vi "Dashboard Main.vi"() -> ()   [LabVIEW 2013]
uses:
  TargetType.ctl
  <vilib>/event_ctls.llb/eventvkey.ctl
  <vilib>/Rock Robotics/WPI/Dashboard/WPI_DashboardLogging Global.vi
  <vilib>/Utility/config.llb/Write Key (String).vi
  <vilib>/Utility/config.llb/Write Key (I32).vi
  <vilib>/Utility/config.llb/NI_LVConfig.lvlib
panel:
  in  "Camera Settings":T1={"Frame Rate"=30, "Compression"=30, "Size"=1} {"Frame Rate" scale=1.0..30.0; "Size" items=["640x480", "320x240", "160x120"]}
  out "Image 3":T2(plugin-control)
  out "Target Info 2":T4(array[cluster])
  in  "Instructions: 3":string="Images:\nUse the tab immediately below to choose the image source. Update the camera settings or the image directory so that you have images or video to test with.\n\nCalibration:\nYou can update Color Component ranges directly, or by clicking and drawing a line on the colored strip in the Image control. The Std Dev multipliers and where the strip is drawn determine the calibration values.\n\nUse Debugging tab to view the result of the color range threshold .\n\nArea Size LImit is used to ignore objects too small or far away to care about.\n\nThe Details tab contains score details for each target and subObject.\n\nCamera Type is used to select lens angles for distance calculation.\n\nVertical strips with no adjacent horizontal strip are identified as \"not hot\" and marked in blue.\nThe numeric scores indicate represent aspect ratio and rectangularity.\n\nWhen both strips are near enough, the pair is identified as \"hot\" and marked in green. Scores\nindicate the left, right, ratio of widths, and vertical positioning.\n\nAny score that falls below cutoff is drawn in red and bounding box is drawn in red."
  in  "Instructions:":string="Images:\nUse the tab immediately below to choose the image source. Update the camera settings or the image directory so that you have images or video to test with.\n\nCalibration:\nYou can update Color Component ranges directly, or by clicking and drawing a line on the colored strip in the Image control. The Std Dev multipliers and where the strip is drawn determine the calibration values.\n\nUse Debugging tab to view the result of the color range threshold .\n\nArea Size LImit is used to ignore objects too small or far away to care about.\n\nThe Details tab contains score details for each target and subObject.\n\nCamera Type is used to select lens angles for distance calculation.\n\nVertical strips with no adjacent horizontal strip are identified as \"not hot\" and marked in blue.\nThe numeric scores indicate represent aspect ratio and rectangularity.\n\nWhen both strips are near enough, the pair is identified as \"hot\" and marked in green. Scores\nindicate the left, right, ratio of widths, and vertical positioning.\n\nAny score that falls below cutoff is drawn in red and bounding box is drawn in red."
  out "Image 2":T2(plugin-control)
  out "Image Message":string="Timeout in Camera Communications"
  in  "Rec Mode":enum32{"Stop", "Record", "Playback"}(radio)
  in  "Dashboard Tab":T5(tab)
  out "MotorSliders R":cluster{"MotorSlide1":dbl, "MotorSlide2":dbl} {"MotorSlide2" scale=-1.0..1.0 scale format="%#_2e"; "MotorSlide1" scale=-1.0..1.0 scale format="%#_2e"}
  out "MotorChart R":cluster{"Numeric":dbl, "Numeric":dbl}(graph)
  out "MotorSliders L":T6 {"MotorSlide4 2" scale=0.0..14.0 scale format="%#_2e"; "MotorSlide2" scale=-1.0..1.0 scale format="%#_2e"; "MotorSlide1" scale=-1.0..1.0 scale format="%#_2e"}
  out "MotorChart L":T7(graph)
  out "JS1 Z":dbl(slide) scale=-1.0..1.0 scale format="%#_2e"
  out "Joystick 1":cluster{"X":dbl, "Y":dbl}[](graph)
  out "JS Buttons 1":T8
  out "JS2 Z":dbl(slide) scale=-1.0..1.0 scale format="%#_2e"
  out "Joystick 2":cluster{"X":dbl, "Y":dbl}[](graph)
  out "JS Buttons 2":T8
  out "Mode":T9(ring)=enum."Auto Disabled"
  out "Camera IP":string
  in  "DB Camera Config":bool
  out "fps":dbl format="%#.1g"
  out "Mbps":dbl format="%#.1g"
  out "Mbps 2":bool
  out "Mask 4":T2(plugin-control)
  out "Goal Hot Or Not?":bool
  in  "Enable":bool
  in  "Color Components":T10={"Hue"={61.0, 119.0}, "Sat"={55.0, 255.0}, "Val"={64.0, 243.0}} {"Val" scale=0.0..255.0; "Sat" scale=0.0..255.0; "Hue" scale=0.0..255.0 scale format="%#_3g"}
  in  "Score Cutoff":dbl(slide)=38.3177570093458 scale=0.0..100.0
  in  "Camera Type":enum16{"206", "1011", "1013"}(ring)=enum."1013"
  in  "Area Size Limit %":dbl=0.06 format="%#_13g"
  in  "Std Devs":cluster{"Hue":dbl, "Sat":dbl, "Val":dbl}={"Hue"=4.0, "Sat"=6.0, "Val"=4.0}
  in  "milliseconds to wait":u32=400
  in  "Auton Routine Names":string[](array[string])
  in  "Routine selected":u16(ring)
  in  "Test Slider":dbl(slide) scale=0.0..100.0 scale format="%#_3g"
  in  "On/Off":bool caption="Solenoid"
  in  "Test Name":u16(ring) items=["Select the test to run...", "Example Test", "-------------------------------", "List of tests is built in robot code.", "Replace with your own automated tests."]
  in  "Test Tree":string(tree)
  in  "Motor":cluster{"Value":dbl, "Enable":bool} {"Value" scale=-1.0..1.0 scale format="%#_3g"}
  out "Progress":T11 {"Test Progress" scale=0.0..100.0}
  in  "Rev/Fwd":cluster{"Forward":bool, "Reverse":bool}
  in  "Test Ring":u16(ring) items=["Auto", "Fixed indoor", "Fixed outdoor 1", "Fixed outdoor 2", "Fixed fluorescent 1", "Fixed fluorescent 2", "Hold current"]
  in  "Listbox":i32(listbox)
  out "Tree":string(tree)
  # "Left"
  # "Front"
  # "Right"
  # "Battery"
  # "Customize by placing controls and indicators here and name to\nmatch Dashboard Variables on robot."
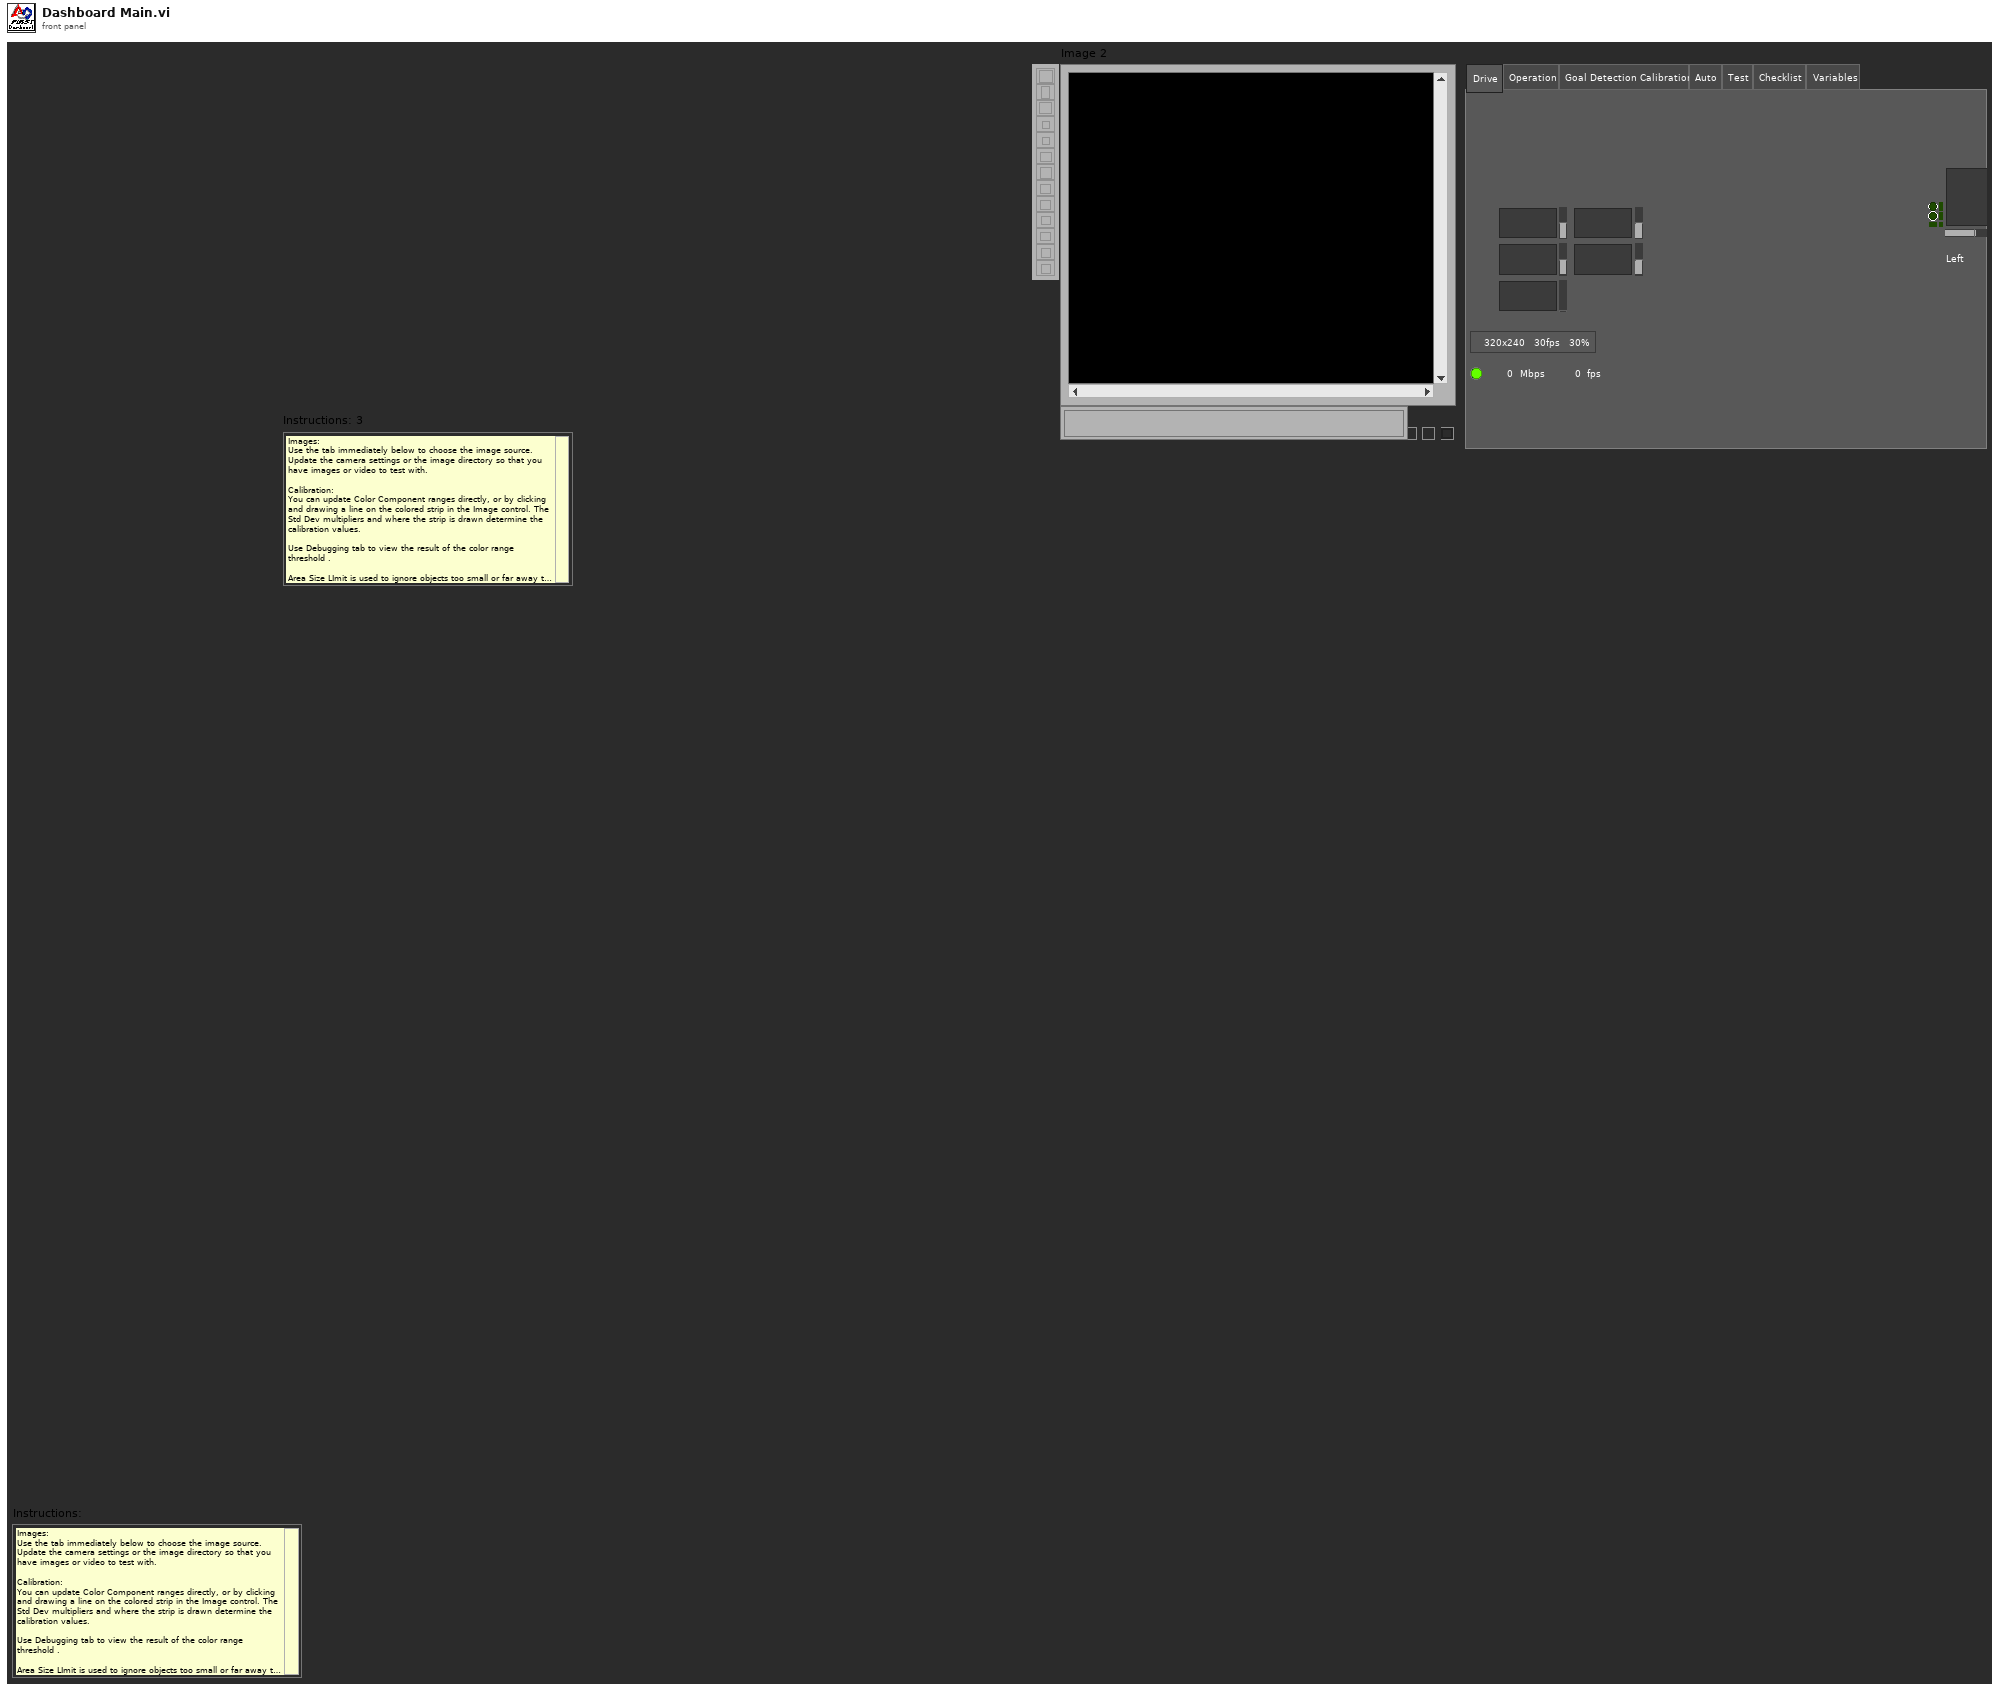
[diagram p1: front panel]
types:
  T1 = cluster{"Frame Rate":i32, "Compression":i32, "Size":u16}
  T2 = typedef "IMAQ Image.ctl" = refnum<image>
  T3 = typedef "TargetType.ctl" = enum16{"Not Hot", "Hot"}
  T4 = cluster{"Scores":cluster{"Total":dbl, "Left":dbl, "Right":dbl, "Ratio":dbl, "Vertical":dbl, "index":i32, "State":T3}, "Verticals":cluster{"Horizontal?":bool, "Aspect Score":dbl, "Rect Score":dbl, cluster{"Left":dbl, "Top":dbl, "Right":dbl, "Bottom":dbl}, "Equiv H":dbl, "Equiv V":dbl}, "Horizontals":cluster{"Horizontal?":bool, "Aspect Score":dbl, "Rect Score":dbl, cluster{"Left":dbl, "Top":dbl, "Right":dbl, "Bottom":dbl}, "Equiv H":dbl, "Equiv V":dbl}, "Distance ft":dbl, "Center":cluster{"X":dbl, "Y":dbl}}[]
  T5 = enum32{"Drive", "Operation", "Goal Detection Calibration", "Auto", "Test", "Checklist", "Variables"}
  T6 = cluster{"MotorSlide1":dbl, "MotorSlide2":dbl, "MotorSlide4 2":dbl}
  T7 = cluster{"Numeric":dbl, "Numeric":dbl, "Battery":sgl}
  T8 = cluster{bool, bool, bool, bool, bool, bool, bool, bool, bool, bool, bool, bool}
  T9 = enum8{"Tele-Op Disabled", "Tele-Op Enabled", "Auto Disabled", "Auto Enabled", "Test Disabled", "Test Enabled", ""}
  T10 = cluster{"Hue":cluster{dbl, dbl}, "Sat":cluster{dbl, dbl}, "Val":cluster{dbl, dbl}}
  T11 = cluster{"Test Progress":u8, "Test Progress Text":string}
  T12 = enum32{"Drive", "Operation", "Vision", "Auto", "Test", "Checklist", "Variables"}
  T13 = typedef "Image Type" = u32
  T14 = cluster{"Horizontal":bool, "Aspect Score":dbl, "Rect Score":dbl, cluster{"Left":dbl, "Top":dbl, "Right":dbl, "Bottom":dbl}, "Equiv H":dbl, "Equiv V":dbl}[]
  T15 = cluster{cluster{dbl, dbl}, cluster{dbl, dbl}, cluster{dbl, dbl}}
  T16 = cluster{"Scores":cluster{"Total":dbl, "Left":dbl, "Right":dbl, "Ratio":dbl, "Vertical":dbl, "index":i32, "State":T3}, "Verticals":cluster{"Horizontal?":bool, "Aspect Score":dbl, "Rect Score":dbl, cluster{"Left":dbl, "Top":dbl, "Right":dbl, "Bottom":dbl}, "Equiv H":dbl, "Equiv V":dbl}, "Horizontals":cluster{"Horizontal?":bool, "Aspect Score":dbl, "Rect Score":dbl, cluster{"Left":dbl, "Top":dbl, "Right":dbl, "Bottom":dbl}, "Equiv H":dbl, "Equiv V":dbl}, "Validated":bool}[]
  T17 = cluster{"Scores":cluster{"Total":dbl, "Left":dbl, "Right":dbl, "Ratio":dbl, "Vertical":dbl, "index":i32, "State":T3}, "Verticals":cluster{"Horizontal?":bool, "Aspect Score":dbl, "Rect Score":dbl, cluster{"Left":dbl, "Top":dbl, "Right":dbl, "Bottom":dbl}, "Equiv H":dbl, "Equiv V":dbl}, "Horizontals":cluster{"Horizontal?":bool, "Aspect Score":dbl, "Rect Score":dbl, cluster{"Left":dbl, "Top":dbl, "Right":dbl, "Bottom":dbl}, "Equiv H":dbl, "Equiv V":dbl}, "Distance (ft)":dbl, "Target Center (-1 to 1)":cluster{"X":dbl, "Y":dbl}}[]
  T18 = cluster{"Scores":cluster{"Total":dbl, "Left":dbl, "Right":dbl, "Ratio":dbl, "Vertical":dbl, "index":i32, "State":T3}, "Verticals":cluster{"Horizontal?":bool, "Aspect Score":dbl, "Rect Score":dbl, cluster{"Left":dbl, "Top":dbl, "Right":dbl, "Bottom":dbl}, "Equiv H":dbl, "Equiv V":dbl}, "Horizontals":cluster{"Horizontal?":bool, "Aspect Score":dbl, "Rect Score":dbl, cluster{"Left":dbl, "Top":dbl, "Right":dbl, "Bottom":dbl}, "Equiv H":dbl, "Equiv V":dbl}, "Distance (ft)":dbl, "Target Center (-1 to 1)":cluster{"X":dbl, "Y":dbl}}
  T19 = typedef "NI_LVConfig.lvlib/Config Data RefNum.ctl" = refnum<k1>
  T20 = cluster{"Digital Inputs":bool[], "Digital Outputs":bool[]}
  T21 = cluster{"Competition mode":bool, "Robot Link":bool, "Autonomous":bool, "Enabled":bool, "E-Stop":bool, "Simulated":bool, "TestMode":bool, "Docked Window":bool}
  T22 = cluster{"Boolean Array[0]":bool, "Boolean Array[1]":bool, "Boolean Array[2]":bool, "Boolean Array[3]":bool, "Boolean Array[4]":bool, "Boolean Array[5]":bool, "Boolean Array[6]":bool, "Boolean Array[7]":bool, "Boolean Array[8]":bool, "Boolean Array[9]":bool, "Boolean Array[10]":bool, "Boolean Array[11]":bool}
  T23 = typedef "eventvkey.ctl" = enum16{"ASCII", "Enter", "Return", "Shift", "Ctrl", "Alt", "Cmd", "Opt", "Caps", "NumLock", "Clear", "Break", "Up", "Down", "Left", "Right", "Insert", "Delete", "Home", "End", "PageUp", "PageDown", "Escape", "Help", "Pause", "ScrollLock", "F1", "F2", "F3", "F4", "F5", "F6", "F7", "F8", "F9", "F10", "F11", "F12", "F13", "F14", "F15", "F16", "F17", "F18", "F19", "F20", "F21", "F22", "F23", "F24", "Play", "VolumeUp", "VolumeDown", "Mute", "Two Byte Char"}
  T24 = cluster{"Image Size":bool, "Image Type":bool, "Pixel Value":bool, "ROI Information":bool, "Zoom Factor":bool}
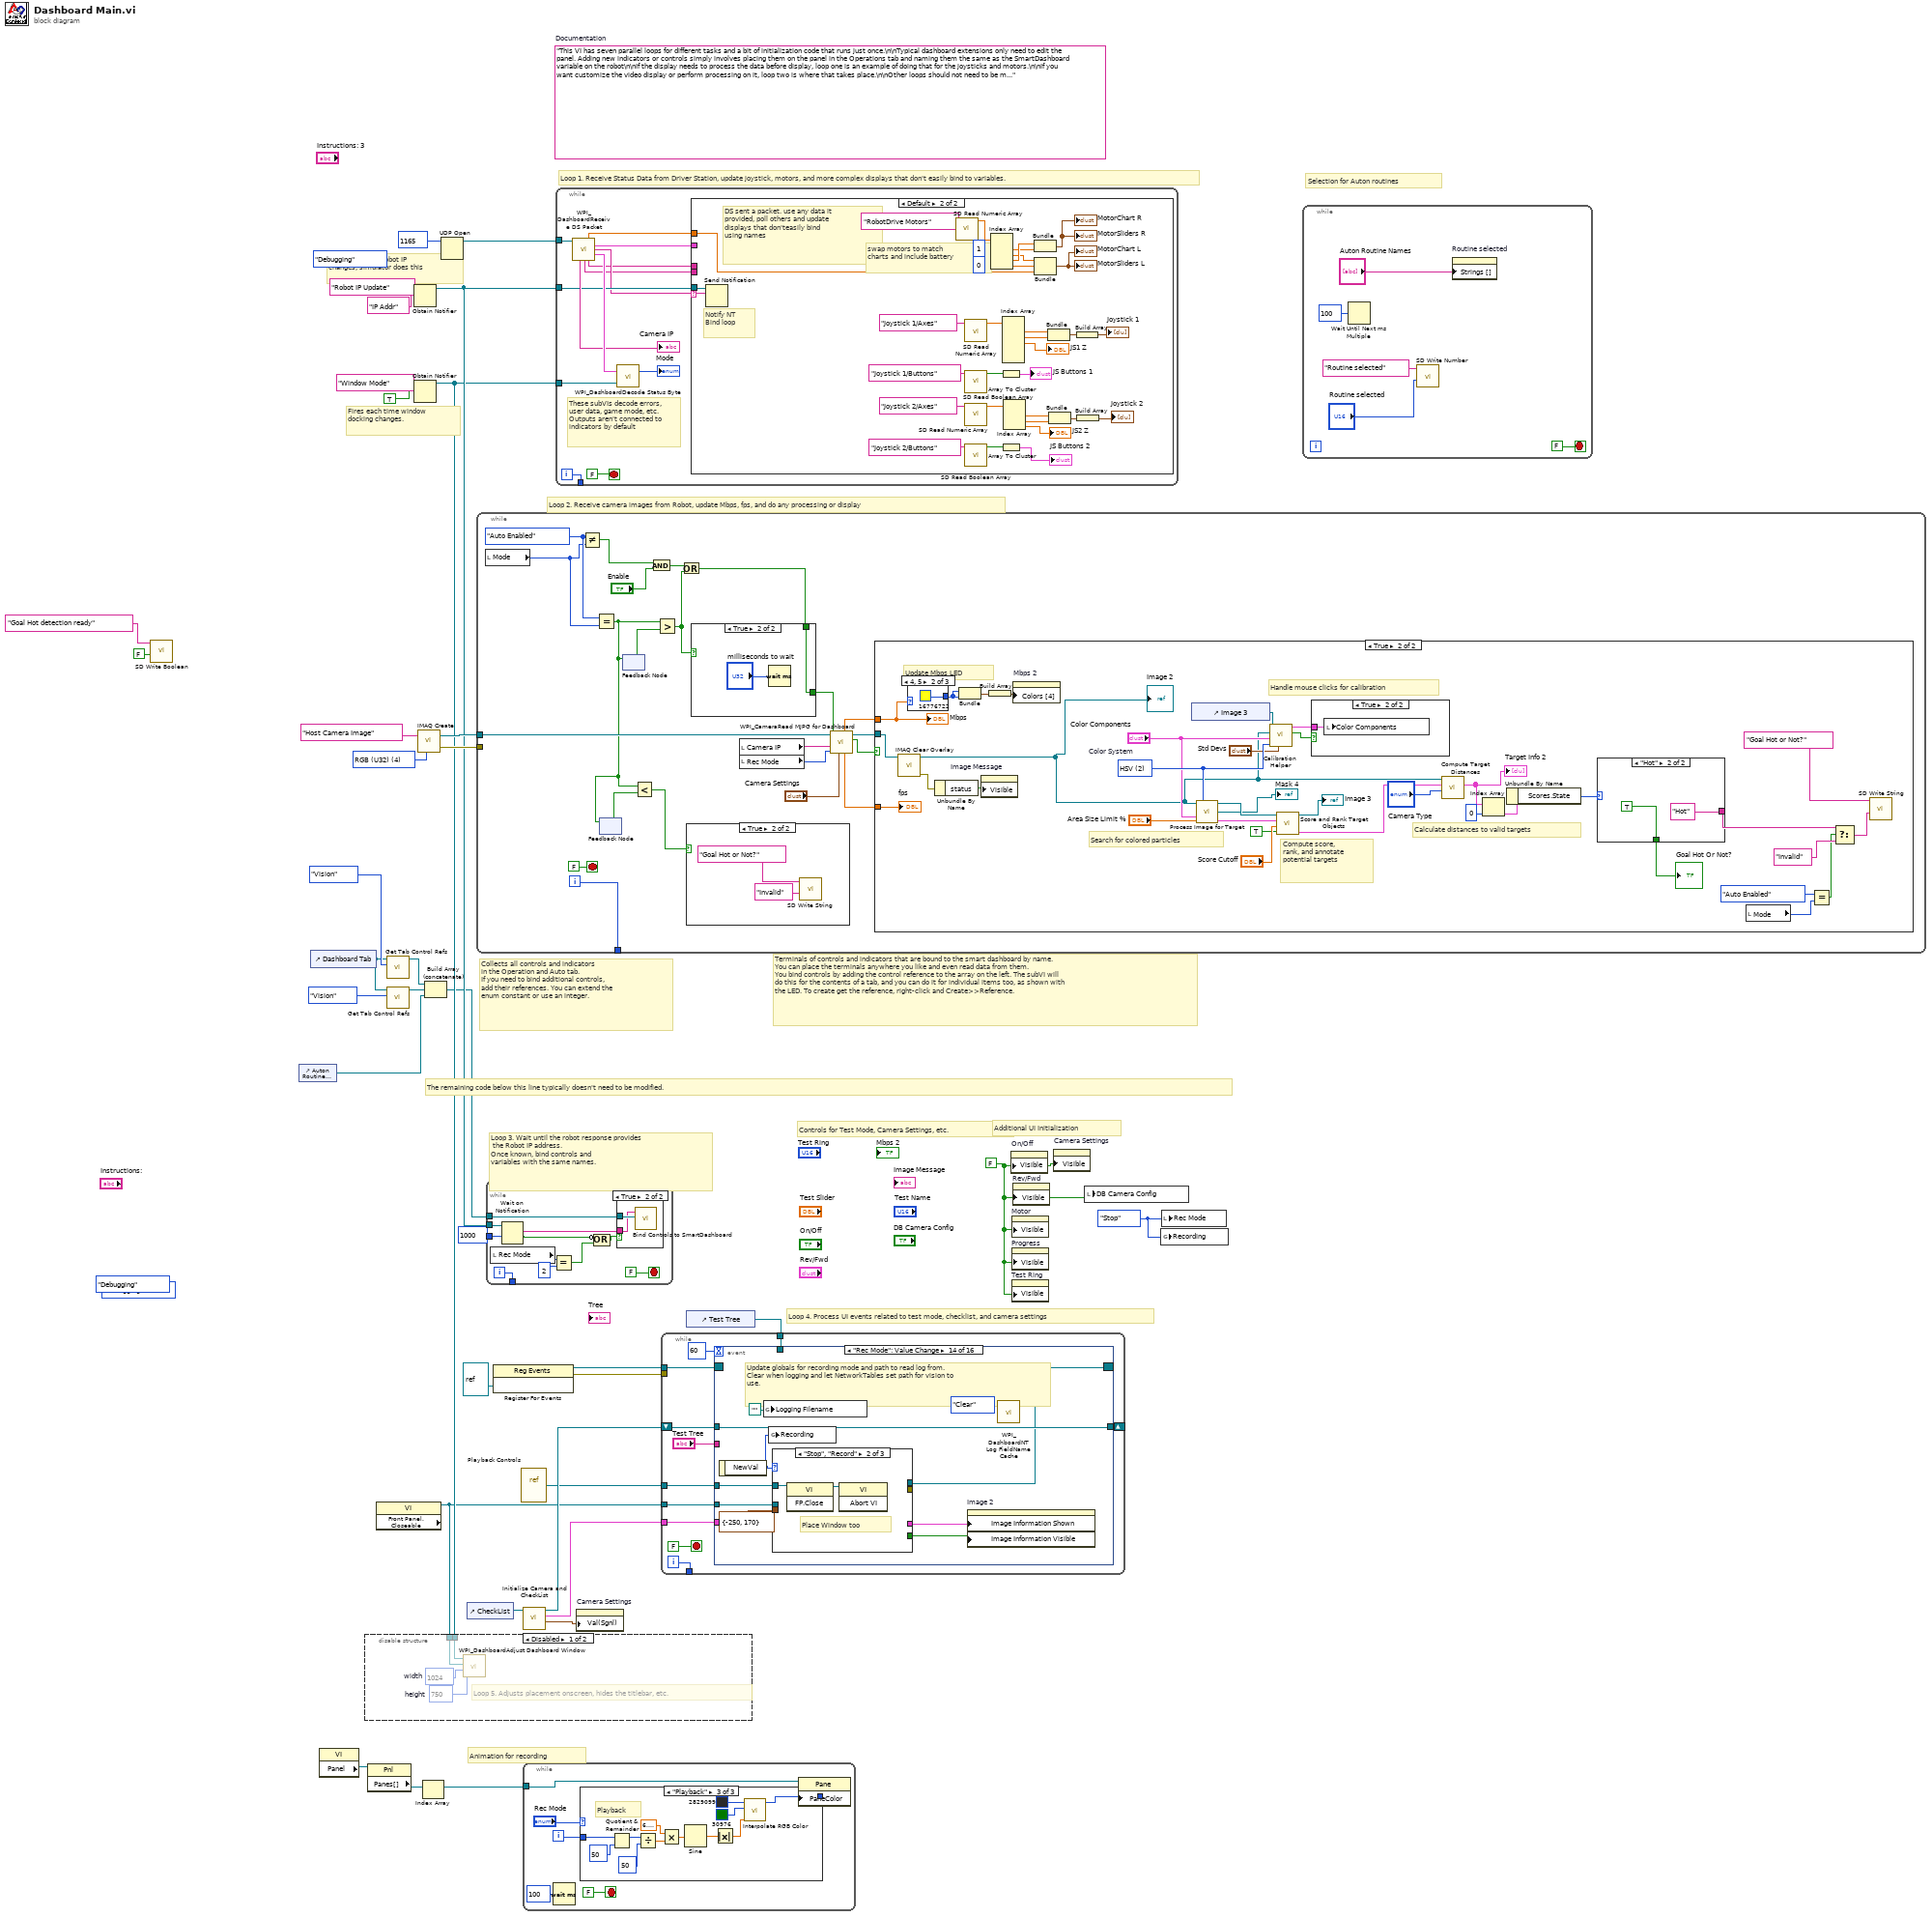
[diagram p0: block diagram]
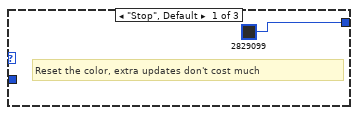
[diagram p3: hidden frame]
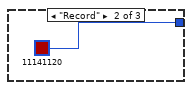
[diagram p4: hidden frame]
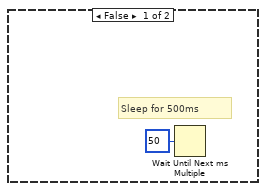
[diagram p8: hidden frame]
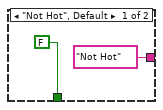
[diagram p9: hidden frame]
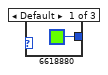
[diagram p11: hidden frame]
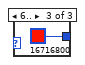
[diagram p12: hidden frame]
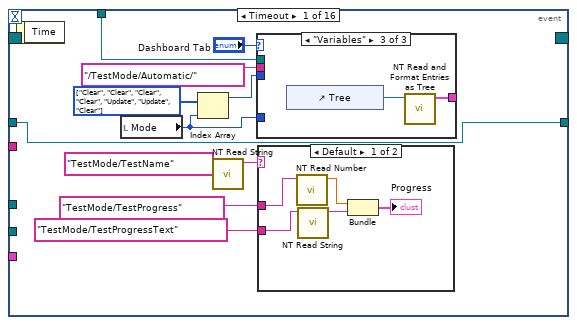
[diagram p13: hidden frame]
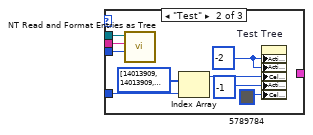
[diagram p15: hidden frame]
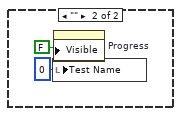
[diagram p16: hidden frame]
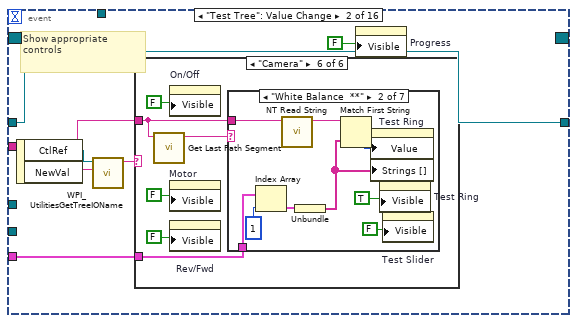
[diagram p17: hidden frame]
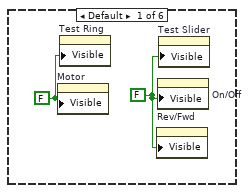
[diagram p18: hidden frame]
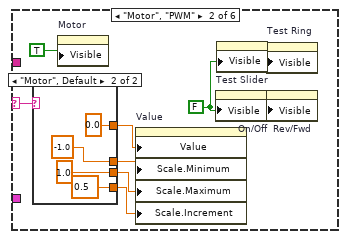
[diagram p19: hidden frame]
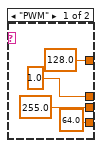
[diagram p20: hidden frame]
diagram:
  (unwired) enum32{"Debugging", "Details"}."Debugging" ("Tabbed Info")
  (unwired) enum32{"Debugging", "Details"}."Debugging" ("Tabbed Info")
  (unwired) enum32{"Debugging", "Details"}."Debugging" ("Tabbed Info")
  w10 = enum32{"Stop", "Record", "Playback"}."Stop" ("Rec Mode")
  w25 = FALSE ("Visible")
  (unwired) "This VI has seven parallel loops for different tasks and a bit of initialization code that runs just once.\n\nTypical dashboard extensions only need to edit the panel. Adding new indicators or controls simply involves placing them on the panel in the Operations tab and naming them the same as the SmartDashboard variable on the robot\n\nIf the display needs to process the data before display, loop one is an example of doing that for the joysticks and motors.\n\nIf you want customize the video display or perform processing on it, loop two is where that takes place.\n\nOther loops should not need to be modified. They are pretty standard, and document the task they perform."  # Documentation
  w35 = T13 4 items=["Grayscale (U8)", "Grayscale (I16)", "Grayscale (SGL)", "Complex (CSG)", "RGB (U32)", "HSL (U32)", "RGB (U64)"] ("Image Type")
  # "Selection for Auton routines"
  # "Controls for Test Mode, Camera Settings, etc."
  # "Additional UI Initialization"
  # "Animation for recording"
  # "Fires each time robot IP\nchanges, simulator does this"
  # "Fires each time window\ndocking changes."
  # "Collects all controls and indicators\nin the Operation and Auto tab.\nIf you need to bind additional controls,\nadd their references. You can extend the\nenum constant or use an integer."
  # "The remaining code below this line typically doesn't need to be modified."
  # "Loop 4. Process UI events related to test mode, checklist, and camera settings"
  # "Terminals of controls and indicators that are bound to the smart dashboard by name.\nYou can place the terminals anywhere you like and even read data from them.\nYou bind controls by adding the control reference to the array on the left. The subVI will\ndo this for the contents of a tab, and you can do it for individual items too, as shown with\nthe LED. To create get the reference, right-click and Create>>Reference."
  # "Loop 3. Wait until the robot response provides\n the Robot IP address.\nOnce known, bind controls and\nvariables with the same names."
  # "Loop 1. Receive Status Data from Driver Station, update joystick, motors, and more complex displays that don't easily bind to variables."
  # "Loop 2. Receive camera images from Robot, update Mbps, fps, and do any processing or display"
  n1 = call <vilib>:"SD Write Boolean.vi"("Boolean"=FALSE, "Name"="Goal Hot detection ready") -> ()  [unwired: 8 in, 2 out]
  n2 = control-ref of="Auton Routine Names"() -> (w3:refnum<vi>)
  n3 = control-ref of="Dashboard Tab"() -> (w8:refnum<vi>)
  n4 = property class="VI"() -> ("Panel"=w19:refnum<vi>)  [unwired: 2 in, 2 out]
  n5 = property class="Pnl"(reference=w19) -> ("Panes[]"=w20:refnum<vi>[])  [unwired: 1 in, 2 out]
  n6 = property class="VI" props=["Front Panel.Closeable"]() -> (reference out=w9:refnum<vi>)  [unwired: 2 in, 2 out]
  n7 = call <vilib>:"Get Tab Control Refs.vi"("Page Index"=T12."Vision" ("Dashboard Tab"), "TabControl in"=w8) -> ("ControlsOnPage"=w6:refnum<vi>[])  [unwired: 9 in]
  n8 = call <vilib>:"Get Tab Control Refs.vi"("Page Index"=T12."Vision" ("Dashboard Tab"), "TabControl in"=w8) -> ("ControlsOnPage"=w7:refnum<vi>[])  [unwired: 9 in]
  n9 = Obtain Notifier(name (unnamed)="Robot IP Update", notification data type="IP Addr" ("name (unnamed)")) -> (notifier out=w29:refnum<notifier>)  [unwired: 2 in, 2 out]
  n10 = Obtain Notifier(name (unnamed)="Window Mode", notification data type=TRUE) -> (notifier out=w12:refnum<notifier>)  [unwired: 2 in, 2 out]
  n11 = disable-structure shown="Disabled" {
    disable-tunnel: w12 -> [w39 _]
    disable-tunnel: w9 -> [w38 _]
    frame Disabled {
      w40 = 750  # height
      w41 = 1024  # width
      # "Loop 5. Adjusts placement onscreen, hides the titlebar, etc."
      n12 = call <vilib>:"WPI_DashboardAdjust Dashboard Window.vi"("height"=w40, "width"=w41, "reference in"=w38, "Notifier in"=w39) -> ()  [unwired: 8 in]
    }
    frame Enabled {
    }
  }
  n13 = call "IMAQ Create"("Image Name"="Host Camera Image", "Image Type"=w35) -> ("New Image"=w33:T2, "error out"=w32:errorcluster)  [unwired: 2 in, 1 out]
  n14 = Index Array(array=w20) -> (element=w18:refnum<vi>)  [unwired: 1 in]
  n15 = Build Array (concatenate)(w6, w7, w3) -> (w5:refnum<vi>[])
  n16 = UDP Open(11:u16 1165 ("port")) -> (port=w36:refnum<k16>)  [unwired: 2 in, 4 out]
  n17 = control-ref of="CheckList"() -> (w11:refnum<vi>)
  n18 = while {
    tunnel: w33 -> [w51]
    tunnel: w32 -> [_]
    tunnel: [w62] -> _
    i -> [w62]
    stop <- FALSE stop-if-true
    w50 = T9."Auto Enabled" ("x")
    n19 = local read "Mode"() -> (w49:T9)
    n20 = Not Equal?(x=w50, y=w49) -> (x != y?=w53:bool)
    n21 = Equal?(x=w50, y=w49) -> (x = y?=w43:bool)
    n22 = feedback #1() -> (w44:bool)  [unwired: 1 in]
    n23 = feedback-in #1(w43) -> ()
    n24 = feedback-in #2(w43) -> ()
    n25 = feedback #2() -> (w48:bool)  [unwired: 1 in]
    n26 = Less?(x=w43, y=w44) -> (x < y?=w42:bool)
    n27 = And(x=w53, y="Enable") -> (x .and. y?=w52:bool)
    n28 = Greater?(x=w43, y=w48) -> (0:w47:bool)
    n29 = Or(x=w52, y=w47) -> (x .or. y?=w45:bool)
    n30 = case shown="True" w42 {
      frame False {
      }
      frame True {
        n31 = call <vilib>:"SD Write String.vi"("String"="Invalid", "Name"="Goal Hot or Not?") -> ()  [unwired: 8 in, 2 out]
      }
    }
    n32 = case shown="True" w47 {
      tunnel: [w66 w67] -> w46
      tunnel: w45 -> [w66 w67]
      frame False {
      }
      frame True {
        n33 = Wait (ms)(milliseconds to wait="milliseconds to wait") -> ()  [unwired: 1 out]
      }
    }
    n34 = local read "Camera IP"() -> (w55:string)
    n35 = local read "Rec Mode"() -> (w56:enum32{"Stop", "Record", "Playback"})
    n36 = call <vilib>:"WPI_CameraRead MJPG for Dashboard.vi"("Camera Settings"="Camera Settings", "Rec Mode"=w56, "Camera IP"=w55, "Enable"=w46, "Refnum in"=w51) -> ("Active"=w60:bool, "Refnum out"=w61:T2, "FPS"=w59:dbl, "Bandwidth (Mbps)"=w58:dbl)  [unwired: 3 in]
    n37 = case shown="True" w60 {
      tunnel: w61 -> [_ w100]
      tunnel: w58 -> [_ w99]
      tunnel: w59 -> [_ w98]
      frame False {
        # "Sleep for 500ms"
        n38 = Wait Until Next ms Multiple(millisecond multiple=u32 50) -> ()  [unwired: 1 out]
      }
      frame True {
        w91 = u16 2 items=["RGB", "HSL", "HSV", "HSI"]  # Color System
        # "Calculate distances to valid targets"
        # "Search for colored particles"
        # "Handle mouse clicks for calibration"
        # "Compute score,\nrank, and annotate\npotential targets"
        # "Update Mbps LED"
        n39 = call "IMAQ Clear Overlay"("Image"=w100) -> ("error out"=w104:errorcluster, "Image Out"=w82:T2)  [unwired: 2 in, 7 out]
        "Image 2" <- w82
        n40 = case shown="4, 5" w99 {
          tunnel: [u32 6618880 ("Color Box") u32 16776722 ("Color Box") u32 16716800 ("Color Box")] -> w101
          frame Default {
          }
          frame 4, 5 {
          }
          frame 6.. {
          }
        }
        n41 = Unbundle By Name(w104) -> ("status"=w105:bool)
        n42 = Bundle("Color Box"=w101, "Color Box"=w101) -> (w103:cluster{"Color Box":u32, "Color Box":u32})  [unwired: 1 out]
        n43 = property on="Image Message" class="Str"("Visible"=w105) -> ()  [unwired: 2 in, 2 out]
        n44 = Build Array(w103) -> (w102:cluster{"Color Box":u32, "Color Box":u32}[])
        n45 = property on="Mbps 2" class="Bool (strict)"("Colors [4]"=w102) -> ()  [unwired: 2 in, 2 out]
        n46 = control-ref of="Image 3"() -> (w79:refnum<vi>)
        n47 = call "Process Image for Target.vi"("Src Image"=w82, "Color Mode"=w91, "Color Components"="Color Components", "Area Cutoff %"="Area Size Limit %") -> ("Src Image Out"=w96:T2, "Threshold"=→"Mask 4":T2, "Particles"=w94:T14)  [unwired: 9 in]
        n48 = call "Calibration Helper.vi"("Std Devs"="Std Devs", "Color Mode"=w91, "Color Components"="Color Components", "Image"=w82, "Image Ctl Refnum"=w79) -> ("Changed"=w87:bool, "output color"=w89:T15)  [unwired: 5 in]
        n49 = call "Score and Rank Target Objects.vi"("Annotate"=TRUE, "Score Limit"="Score Cutoff", "Particles"=w94, "Image in"=w96) -> ("Target Info"=w93:T16, "Annotated Image"=→"Image 3":T2)  [unwired: 6 in]
        n50 = case shown="True" w87 {
          tunnel: w89 -> [_ w110]
          frame False {
          }
          frame True {
            n51 = local write "Color Components"(w110) -> ()
          }
        }
        n52 = call "Compute Target Distances.vi"("Camera Type"="Camera Type", "Target Info"=w93, "Image in"=w82) -> ("Target Info"=w80:T17)  [unwired: 6 in, 2 out]
        "Target Info 2" <- w80
        n53 = Index Array(array=w80, index=0) -> (element=w84:T18)
        n54 = Unbundle By Name(w84) -> ("Scores.State"=w83:T3)
        n55 = case shown="\"Hot\"" w83 {
          tunnel: [FALSE TRUE] -> w76
          tunnel: ["Not Hot" "Hot"] -> w75
          frame "Not Hot", Default {
          }
          frame "Hot" {
          }
        }
        "Goal Hot Or Not?" <- w76
        n56 = local read "Mode"() -> (w72:T9)
        n57 = Equal?(x=T9."Auto Enabled", y=w72) -> (x = y?=w70:bool)
        n58 = Select(t=w75, s=w70, f="Invalid") -> (s? t:f=w74:string)
        n59 = call <vilib>:"SD Write String.vi"("String"=w74, "Name"="Goal Hot or Not?") -> ()  [unwired: 8 in, 2 out]
        "Mbps" <- w99
        "fps" <- w98
      }
    }
  }
  n60 = while {
    tunnel: w5 -> [w124]
    tunnel: w29 -> [w122]
    tunnel: [w120] -> _
    tunnel: u32 1000 ("milliseconds to wait") -> [w119]
    i -> [w120]
    stop <- FALSE stop-if-true
    n61 = local read "Rec Mode"() -> (w115:enum32{"Stop", "Record", "Playback"})
    n62 = Wait on Notification(notifier=w122, timeout in ms (-1)=w119) -> (notification=w121:string, timed out?=w117:bool)  [unwired: 2 in, 2 out]
    n63 = Equal?(x=w115, y=u16 2 ("Rec Mode")) -> (x = y?=w116:bool)
    n64 = Compound Arithmetic op=OR(invert w117, w116) -> (w118:bool)
    n65 = case shown="True" w118 {
      tunnel: w124 -> [_ w126]
      tunnel: w121 -> [_ w125]
      frame False {
      }
      frame True {
        n66 = call <vilib>:"Bind Controls to SmartDashboard.vi"("Bound Control Refs"=w126, "Server IP Address"=w125) -> ()  [unwired: 10 in]
      }
    }
  }
  n67 = register-events(refnum<vi> refnum) -> (reference out=w16:refnum<event-registration>, error out=w15:errorcluster)  [unwired: 2 in]
  n68 = vi-ref "Playback Controls.vi"() -> (w17:refnum<vi>)
  n69 = while {
    tunnel: w18 -> [w128]
    i -> [w131]
    stop <- FALSE stop-if-true
    n70 = Wait (ms)(milliseconds to wait=u32 100) -> ()  [unwired: 1 out]
    n71 = case shown="\"Playback\"" "Rec Mode" {
      tunnel: w131 -> [_ _ w146]
      tunnel: [u32 2829099 ("Base Color") u32 11141120 ("Target Color") w135] -> w127
      frame "Stop", Default {
        # "Reset the color, extra updates don't cost much"
      }
      frame "Record" {
      }
      frame "Playback" {
        # "Playback"
        n72 = Quotient & Remainder(x=w146, y=u32 50 ("milliseconds to wait")) -> (x-y*floor(x/y)=w142:u32)  [unwired: 1 out]
        n73 = Divide(x=w142, y=u32 50 ("milliseconds to wait")) -> (x/y=w139:dbl)
        n74 = Multiply(x=6.283185307179586, y=w139) -> (x*y=w144:dbl)
        n75 = Sine(x=w144) -> (sin(x)=w143:dbl)
        n76 = Absolute Value(x=w143) -> (abs(x)=w136:dbl)
        n77 = call "Interpolate RGB Color.vi"("Proportion"=w136, "Target Color"=u32 30976, "Base Color"=u32 2829099) -> ("Result Color"=w135:u32)  [unwired: 8 in]
      }
    }
    n78 = property class="Pane"(reference=w128, "PaneColor"=w127) -> ()  [unwired: 1 in, 2 out]
  }
  n79 = call "Initialize Camera and CheckList.vi"("ListBox in"=w11) -> ("Cluster"=w23:cluster{"value":i32, "value":i32, "index":i32}, "Array"=w24:cluster{string[]}[], "File Refnum"=w22:T19)  [unwired: 8 in]
  n80 = while {
    tunnel: w36 -> [w157]
    tunnel: w29 -> [w152]
    tunnel: w12 -> [w156]
    tunnel: [w153] -> _
    i -> [w153]
    stop <- FALSE stop-if-true
    # "These subVIs decode errors, user data, game mode, etc.\nOutputs aren't connected to indicators by default"
    n81 = call <vilib>:"WPI_DashboardReceive DS Packet.vi"("Recv Socket"=w157) -> ("Battery"=w147:sgl, "Driver Station"=w148:T20, "Robot IP Address"=w151:string, "Status"=w158:T21, "Camera IP Address"=→"Camera IP":string, "Low Priority User Data"=w150:string, "High Priority User Data"=w149:string)  [unwired: 1 in, 7 out]
    n82 = call <vilib>:"WPI_DashboardDecode Status Byte.vi"("Window Mode Notifier"=w156, "Status"=w158) -> ("Mode"=→"Mode":T9)  [unwired: 1 out]
    n83 = case shown="Default" w151 {
      selector: w151 -> [_ w170]
      tunnel: w152 -> [_ w171]
      tunnel: w150 -> [_ _]
      tunnel: w149 -> [_ _]
      tunnel: w148 -> [_ _]
      tunnel: w147 -> [_ w169]
      frame "0.0.0.0" {
        # "DS not sending packets, or no robot exists yet.\nDon't poll the variables"
      }
      frame Default {
        # "Notify NT\nBind loop"
        # "DS sent a packet. use any data it\nprovided, poll others and update\ndisplays that don'teasily bind\nusing names"
        # "swap motors to match\ncharts and include battery"
        n84 = Send Notification(notification=w170, notifier=w171) -> ()  [unwired: 1 in, 2 out]
        n85 = call <vilib>:"SD Read Numeric Array.vi"("Name"="RobotDrive Motors") -> ("Numeric Array"=w168:dbl[])  [unwired: 8 in, 2 out]
        n86 = call <vilib>:"SD Read Numeric Array.vi"("Name"="Joystick 1/Axes") -> ("Numeric Array"=w187:dbl[])  [unwired: 8 in, 2 out]
        n87 = call <vilib>:"SD Read Boolean Array.vi"("Name"="Joystick 1/Buttons") -> ("Boolean Array"=w189:bool[])  [unwired: 8 in, 2 out]
        n88 = call <vilib>:"SD Read Numeric Array.vi"("Name"="Joystick 2/Axes") -> ("Numeric Array"=w181:dbl[])  [unwired: 8 in, 2 out]
        n89 = call <vilib>:"SD Read Boolean Array.vi"("Name"="Joystick 2/Buttons") -> ("Boolean Array"=w180:bool[])  [unwired: 8 in, 2 out]
        n90 = Index Array(array=w168, index #1=1, index #4=0) -> (element #1=w164:dbl, element #2=w163:dbl, element #3=w165:dbl, element #4=w160:dbl)  [unwired: 2 in]
        n91 = Array To Cluster(array=w189) -> (cluster=→"JS Buttons 1":T22)
        n92 = Array To Cluster(array=w180) -> (cluster=→"JS Buttons 2":T22)
        n93 = Index Array(array=w187) -> (element #1=w184:dbl, element #2=w185:dbl, element #3=→"JS1 Z":dbl)  [unwired: 6 in, 3 out]
        n94 = Index Array(array=w181) -> (element #1=w176:dbl, element #2=w175:dbl, element #3=→"JS2 Z":dbl)  [unwired: 3 in]
        n95 = Bundle("Numeric"=w165, "Numeric"=w164) -> (→"MotorChart R" →"MotorSliders R":cluster{"Numeric":dbl, "Numeric":dbl})  [unwired: 1 in]
        n96 = Bundle("Numeric"=w163, "Numeric"=w160, "Battery"=w169) -> (→"MotorChart L" →"MotorSliders L":T7)  [unwired: 1 in]
        n97 = Bundle("Numeric"=w184, "Numeric"=w185) -> (w183:cluster{"Numeric":dbl, "Numeric":dbl})  [unwired: 1 in]
        n98 = Bundle("Numeric"=w176, "Numeric"=w175) -> (w177:cluster{"Numeric":dbl, "Numeric":dbl})  [unwired: 1 in]
        n99 = Build Array(w183) -> (→"Joystick 1":cluster{"Numeric":dbl, "Numeric":dbl}[])
        n100 = Build Array(w177) -> (→"Joystick 2":cluster{"Numeric":dbl, "Numeric":dbl}[])
      }
    }
  }
  n101 = property on="Camera Settings" class="Clust (strict)"("Val(Sgnl)"=w23) -> ()  [unwired: 2 in, 2 out]
  n102 = control-ref of="Test Tree"() -> (w21:refnum<vi>)
  n103 = while {
    tunnel: w24 -> [w200]
    shift-right: [w199] -> _
    shift-left: w22 -> [w198]
    tunnel: [w197] -> _
    tunnel: w21 -> [w196]
    tunnel: w17 -> [w195]
    tunnel: w16 -> [w194]
    tunnel: w15 -> [_]
    tunnel: w9 -> [w193]
    i -> [w197]
    stop <- FALSE stop-if-true
    n104 = event shown="[13] \"Rec Mode\": Value Change" {
      selector: w194 -> [_ _ _ _ _ _ _ _ _ _ _ _ _ _ _ _]
      dyn-events: [_ _ _ _ _ _ _ _ _ _ _ _ _ w438 _ _] -> _
      timeout: u32 60 ("milliseconds to wait") -> [_ _ _ _ _ _ _ _ _ _ _ _ _ _ _ _]
      tunnel: w196 -> [w210 _ _ _ _ _ _ _ _ _ _ _ _ _ _ _]
      tunnel: "Test Tree" -> [_ _ _ _ _ _ _ _ w407 w415 w417 w421 w429 _ _ _]
      tunnel: w200 -> [_ w234 _ _ _ _ w371 w401 _ _ _ _ _ _ _ _]
      tunnel: [w204 w233 w332 w337 w345 w357 w370 w394 w406 w413 w416 w420 w428 w440 w454 w455] -> w199
      tunnel: w198 -> [w204 w233 w332 w337 w345 w357 w369 w394 w406 w413 w416 w420 w428 w440 w454 w455]
      tunnel: w195 -> [_ _ _ _ _ _ _ _ _ _ _ _ _ w441 _ w458]
      tunnel: w193 -> [_ _ _ _ _ _ _ _ _ _ _ _ _ w436 _ _]
      event Timeout {
        w209 = enum16{"Update", "Clear"}[] [enum."Clear", enum."Clear", enum."Clear", enum."Clear", enum."Update", enum."Update", enum."Clear"] items=["Update", "Clear"]
        n105 = event-data() -> ()  [unwired: 1 in, 1 out]
        n106 = local read "Mode"() -> (w207:T9)
        n107 = Index Array(array=w209, index=w207) -> (element=w208:enum16{"Update", "Clear"})
        n108 = call <vilib>:"NT Read String.vi"("Name"="TestMode/TestName") -> ("String"=w213:string)  [unwired: 9 in, 1 out]
        n109 = case shown="\"Variables\"" "Dashboard Tab" {
          tunnel: w210 -> [_ w223 _]
          tunnel: "/TestMode/Automatic/" ("Name Pattern") -> [_ w222 _]
          tunnel: w208 -> [_ w221 _]
          tunnel: w207 -> [_ w219 _]
          tunnel: [_ _ w225] -> _
          frame "Operation", Default {
          }
          frame "Test" {
            w218 = -2 ("Active Item:Row Number")
            n110 = call <vilib>:"NT Read and Format Entries as Tree.vi"("Operation"=w221, "Name Pattern"=w222, "Tree Refnum"=w223) -> ()  [unwired: 7 in, 2 out]
            n111 = Index Array(array=u32[] [14013909, 14013909, 14013909, 14013909, 14013909, 16777215, 14013909], index=w219) -> (element=w217:u32)
            n112 = property on="Test Tree" class="Tree (strict)"("Active Item Row Number"=w218, "ActiveColNum"=w218, "CellBG"=w217, "Active Item Row Number"=-1 ("Active Item:Row Number"), "CellBG"=u32 5789784 ("Color Box")) -> ()  [unwired: 2 in, 2 out]
          }
          frame "Variables" {
            n113 = control-ref of="Tree"() -> (w224:refnum<vi>)
            n114 = call <vilib>:"NT Read and Format Entries as Tree.vi"("Tree Refnum"=w224) -> ("Formatted Strings"=w225:cluster{"Name":string, "Value":string}[])  [unwired: 9 in, 1 out]
          }
        }
        n115 = case shown="Default" w213 {
          tunnel: "TestMode/TestProgress" ("Name") -> [w227 _]
          tunnel: "TestMode/TestProgressText" ("Name") -> [w226 _]
          frame Default {
            n116 = call <vilib>:"NT Read Number.vi"("Name"=w227) -> ("Numeric"=w228:dbl)  [unwired: 9 in, 1 out]
            n117 = call <vilib>:"NT Read String.vi"("Name"=w226) -> ("String"=w229:string)  [unwired: 9 in, 1 out]
            n118 = Bundle("Numeric"=w228, "String"=w229) -> (→"Progress":cluster{"Numeric":dbl, "String":string})  [unwired: 1 in]
          }
          frame "" {
            n119 = local write "Test Name"(u16 0) -> ()
            n120 = property on="Progress" class="Clust (strict)"("Visible"=FALSE) -> ()  [unwired: 2 in, 2 out]
          }
        }
      }
      event "Test Tree": Value Change {
        # "Show appropriate\ncontrols"
        n121 = event-data() -> ("CtlRef"=w237:refnum<vi>, "NewVal"=w235:string)  [unwired: 1 in]
        n122 = call <vilib>:"WPI_UtilitiesGetTreeIOName.vi"("NewVal"=w235, "TreeControl in"=w237) -> ("I/O Name"=w238:string)  [unwired: 9 in]
        n123 = case shown="\"Camera\"" w238 {
          selector: w238 -> [_ w245 _ w263 w272 _]
          tunnel: w235 -> [_ _ w260 w262 _ w279]
          tunnel: w234 -> [_ _ _ _ _ w278]
          frame Default {
            w240 = FALSE ("Visible")
            w239 = FALSE ("Visible")
            n124 = property on="Motor" class="Clust (strict)"("Visible"=w239) -> ()  [unwired: 2 in, 2 out]
            n125 = property on="Test Ring" class="Ring (strict)"("Visible"=w239) -> ()  [unwired: 2 in, 2 out]
            n126 = property on="Rev/Fwd" class="Clust (strict)"("Visible"=w240) -> ()  [unwired: 2 in, 2 out]
            n127 = property on="On/Off" class="Bool (strict)"("Visible"=w240) -> ()  [unwired: 2 in, 2 out]
            n128 = property on="Test Slider" class="Slide (strict)"("Visible"=w240) -> ()  [unwired: 2 in, 2 out]
          }
          frame "Motor", "PWM" {
            w246 = FALSE ("Visible")
            n129 = case shown="\"Motor\", Default" w245 {
              tunnel: [1.0 ("Value") -1.0 ("Value")] -> w244
              tunnel: [255.0 ("Value") 1.0 ("Value")] -> w243
              tunnel: [128.0 ("Value") 0.0 ("Value")] -> w242
              tunnel: [64.0 ("Value") 0.5 ("Value")] -> w241
              frame "PWM" {
              }
              frame "Motor", Default {
              }
            }
            n130 = property on="Motor" class="Clust (strict)"("Visible"=TRUE) -> ()  [unwired: 2 in, 2 out]
            n131 = property on="Value" class="Slide (strict)"("Value"=w242, "Scale.Minimum"=w244, "Scale.Maximum"=w243, "Scale.Increment"=w241) -> ()  [unwired: 2 in, 2 out]
            n132 = property on="On/Off" class="Bool (strict)"("Visible"=w246) -> ()  [unwired: 2 in, 2 out]
            n133 = property on="Test Slider" class="Slide (strict)"("Visible"=w246) -> ()  [unwired: 2 in, 2 out]
            n134 = property on="Test Ring" class="Ring (strict)"("Visible"=w246) -> ()  [unwired: 2 in, 2 out]
            n135 = property on="Rev/Fwd" class="Clust (strict)"("Visible"=w246) -> ()  [unwired: 2 in, 2 out]
          }
          frame "Servo" {
            w258 = FALSE ("Visible")
            n136 = call <vilib>:"NT Read Number.vi"("Name"=w260) -> ("Numeric"=w259:dbl)  [unwired: 9 in, 1 out]
            n137 = property on="Test Slider" class="Slide (strict)"("Visible"=TRUE, "Scale.Maximum"=170.0 ("Scale.Range:Maximum")) -> ()  [unwired: 2 in, 2 out]
            n138 = local write "Test Slider"(w259) -> ()
            n139 = property on="Motor" class="Clust (strict)"("Visible"=w258) -> ()  [unwired: 2 in, 2 out]
            n140 = property on="Rev/Fwd" class="Clust (strict)"("Visible"=w258) -> ()  [unwired: 2 in, 2 out]
            n141 = property on="On/Off" class="Bool (strict)"("Visible"=w258) -> ()  [unwired: 2 in, 2 out]
            n142 = property on="Test Ring" class="Ring (strict)"("Visible"=w258) -> ()  [unwired: 2 in, 2 out]
          }
          frame "Relay", "Solenoid" {
            w261 = FALSE ("Visible")
            n143 = property on="Motor" class="Clust (strict)"("Visible"=w261) -> ()  [unwired: 2 in, 2 out]
            n144 = property on="Test Slider" class="Slide (strict)"("Visible"=w261) -> ()  [unwired: 2 in, 2 out]
            n145 = Search and Replace String(input string=w262, search string="/Value  **", replace string="/Direction") -> (result string=w268:string)  [unwired: 5 in, 3 out]
            n146 = property on="Test Ring" class="Ring (strict)"("Visible"=w261) -> ()  [unwired: 2 in, 2 out]
            n147 = call <vilib>:"NT Read String.vi"("Name"=w268) -> ("String"=w266:string)  [unwired: 9 in, 1 out]
            n148 = Equal?(x="Both directions", y=w266) -> (x = y?=w264:bool)
            n149 = Not(x=w264) -> (.not. x?=w265:bool)
            n150 = property on="Rev/Fwd" class="Clust (strict)"("Visible"=w264) -> ()  [unwired: 2 in, 2 out]
            n151 = property on="On/Off" class="Bool (strict)"("Visible"=w265, "Caption.Text"=w263) -> ()  [unwired: 2 in, 2 out]
          }
          frame "Compressor", "Digital Out" {
            w271 = FALSE ("Visible")
            # "Get direction and finish"
            n152 = property on="Motor" class="Clust (strict)"("Visible"=w271) -> ()  [unwired: 2 in, 2 out]
            n153 = property on="Test Slider" class="Slide (strict)"("Visible"=w271) -> ()  [unwired: 2 in, 2 out]
            n154 = property on="Test Ring" class="Ring (strict)"("Visible"=w271) -> ()  [unwired: 2 in, 2 out]
            n155 = property on="On/Off" class="Bool (strict)"("Visible"=TRUE, "Caption.Text"=w272) -> ()  [unwired: 2 in, 2 out]
            n156 = property on="Rev/Fwd" class="Clust (strict)"("Visible"=FALSE) -> ()  [unwired: 2 in, 2 out]
          }
          frame "Camera" {
            n157 = call <vilib>:"Get Last Path Segment.vi"("String in"=w279) -> ("String out"=w280:string)  [unwired: 10 in]
            n158 = property on="On/Off" class="Bool (strict)"("Visible"=FALSE) -> ()  [unwired: 2 in, 2 out]
            n159 = property on="Motor" class="Clust (strict)"("Visible"=FALSE) -> ()  [unwired: 2 in, 2 out]
            n160 = property on="Rev/Fwd" class="Clust (strict)"("Visible"=FALSE) -> ()  [unwired: 2 in, 2 out]
            n161 = case shown="\"White Balance  **\"" w280 {
              tunnel: w279 -> [w286 w295 w304 w313 w322 _ w328]
              tunnel: w278 -> [w284 w292 w301 w310 w319 _ _]
              frame "Size  **" {
                n162 = Index Array(array=w284) -> (element=w283:cluster{string[]})  [unwired: 1 in]
                n163 = call <vilib>:"NT Read String.vi"("Name"=w286) -> ("String"=w285:string)  [unwired: 9 in, 1 out]
                n164 = Unbundle(w283) -> (w281:string[])
                n165 = Match First String(2:w281, 3:w285) -> (0:w282:i32)  [unwired: 1 out]
                n166 = property on="Test Ring" class="Ring (strict)"("Value"=w282, "Strings []"=w281) -> ()  [unwired: 2 in, 2 out]
                n167 = property on="Test Ring" class="Ring (strict)"("Visible"=TRUE) -> ()  [unwired: 2 in, 2 out]
                n168 = property on="Test Slider" class="Slide (strict)"("Visible"=FALSE) -> ()  [unwired: 2 in, 2 out]
              }
              frame "White Balance  **" {
                n169 = Index Array(array=w292, index=1) -> (element=w293:cluster{string[]})
                n170 = call <vilib>:"NT Read String.vi"("Name"=w295) -> ("String"=w294:string)  [unwired: 9 in, 1 out]
                n171 = Unbundle(w293) -> (w290:string[])
                n172 = Match First String(2:w290, 3:w294) -> (0:w289:i32)  [unwired: 1 out]
                n173 = property on="Test Ring" class="Ring (strict)"("Value"=w289, "Strings []"=w290) -> ()  [unwired: 2 in, 2 out]
                n174 = property on="Test Ring" class="Ring (strict)"("Visible"=TRUE) -> ()  [unwired: 2 in, 2 out]
                n175 = property on="Test Slider" class="Slide (strict)"("Visible"=FALSE) -> ()  [unwired: 2 in, 2 out]
              }
              frame "Exposure  **" {
                n176 = Index Array(array=w301, index=2) -> (element=w302:cluster{string[]})
                n177 = call <vilib>:"NT Read String.vi"("Name"=w304) -> ("String"=w303:string)  [unwired: 9 in, 1 out]
                n178 = Unbundle(w302) -> (w298:string[])
                n179 = Match First String(2:w298, 3:w303) -> (0:w299:i32)  [unwired: 1 out]
                n180 = property on="Test Ring" class="Ring (strict)"("Value"=w299, "Strings []"=w298) -> ()  [unwired: 2 in, 2 out]
                n181 = property on="Test Ring" class="Ring (strict)"("Visible"=TRUE) -> ()  [unwired: 2 in, 2 out]
                n182 = property on="Test Slider" class="Slide (strict)"("Visible"=FALSE) -> ()  [unwired: 2 in, 2 out]
              }
              frame "Exposure Priority  **" {
                n183 = Index Array(array=w310, index=3) -> (element=w311:cluster{string[]})
                n184 = call <vilib>:"NT Read String.vi"("Name"=w313) -> ("String"=w312:string)  [unwired: 9 in, 1 out]
                n185 = Unbundle(w311) -> (w307:string[])
                n186 = Match First String(2:w307, 3:w312) -> (0:w308:i32)  [unwired: 1 out]
                n187 = property on="Test Ring" class="Ring (strict)"("Value"=w308, "Strings []"=w307) -> ()  [unwired: 2 in, 2 out]
                n188 = property on="Test Ring" class="Ring (strict)"("Visible"=TRUE) -> ()  [unwired: 2 in, 2 out]
                n189 = property on="Test Slider" class="Slide (strict)"("Visible"=FALSE) -> ()  [unwired: 2 in, 2 out]
              }
              frame "Color Enable  **" {
                n190 = Index Array(array=w319, index=4) -> (element=w320:cluster{string[]})
                n191 = call <vilib>:"NT Read String.vi"("Name"=w322) -> ("String"=w321:string)  [unwired: 9 in, 1 out]
                n192 = Unbundle(w320) -> (w316:string[])
                n193 = Match First String(2:w316, 3:w321) -> (0:w317:i32)  [unwired: 1 out]
                n194 = property on="Test Ring" class="Ring (strict)"("Value"=w317, "Strings []"=w316) -> ()  [unwired: 2 in, 2 out]
                n195 = property on="Test Ring" class="Ring (strict)"("Visible"=TRUE) -> ()  [unwired: 2 in, 2 out]
                n196 = property on="Test Slider" class="Slide (strict)"("Visible"=FALSE) -> ()  [unwired: 2 in, 2 out]
              }
              frame Default {
                n197 = property on="Test Ring" class="Ring (strict)"("Visible"=FALSE) -> ()  [unwired: 2 in, 2 out]
                n198 = property on="Test Slider" class="Slide (strict)"("Visible"=FALSE) -> ()  [unwired: 2 in, 2 out]
              }
              frame "Brightness  **", "Color Level  **", "Compression  **", "FPS  **", "Sharpness  **" {
                n199 = call <vilib>:"NT Read Number.vi"("Name"=w328) -> ("Numeric"=w327:dbl)  [unwired: 9 in, 1 out]
                n200 = local write "Test Slider"(w327) -> ()
                n201 = property on="Test Slider" class="Slide (strict)"("Visible"=TRUE, "Scale.Maximum"=100.0 ("Scale.Range:Maximum")) -> ()  [unwired: 2 in, 2 out]
                n202 = property on="Test Ring" class="Ring (strict)"("Visible"=FALSE) -> ()  [unwired: 2 in, 2 out]
              }
            }
          }
        }
        n203 = property on="Progress" class="Clust (strict)"("Visible"=FALSE) -> ()  [unwired: 2 in, 2 out]
      }
      event "Test Name": Mouse Enter {
        # "Populate the ring with the list of tests"
        n204 = event-data() -> ()  [unwired: 1 in, 1 out]
        n205 = call <vilib>:"NT Read String Array.vi"("Name"="TestMode/TestList") -> ("String Array"=w336:string[])  [unwired: 9 in, 1 out]
        n206 = Build Array (concatenate)("Select the test to run...", w336) -> (w335:string[])
        n207 = property on="Test Name" class="Ring (strict)"("Strings []"=w335) -> ()  [unwired: 2 in, 2 out]
      }
      event "Test Name": Value Change {
        w338 = FALSE ("Visible")
        # "Tell the robot the test name to run"
        n208 = event-data() -> ("NewVal"=w342:u16)  [unwired: 1 in]
        n209 = property on="Test Name" class="Ring (strict)"() -> ("Strings []"=w343:string[])  [unwired: 2 in, 2 out]
        n210 = local write "Progress"(T11 {"Test Progress"=0, "Test Progress Text"=""} ("Progress")) -> ()
        n211 = Index Array(array=w343, index=w342) -> (element=w341:string)
        n212 = call <vilib>:"NT Write String.vi"("String"=w341, "Name"="TestMode/TestName") -> ()  [unwired: 9 in, 1 out]
        n213 = property on="Progress" class="Clust (strict)"("Visible"=TRUE) -> ()  [unwired: 2 in, 2 out]
        n214 = property on="Motor" class="Clust (strict)"("Visible"=w338) -> ()  [unwired: 2 in, 2 out]
        n215 = property on="Test Slider" class="Slide (strict)"("Visible"=w338) -> ()  [unwired: 2 in, 2 out]
        n216 = property on="On/Off" class="Bool (strict)"("Visible"=w338) -> ()  [unwired: 2 in, 2 out]
        n217 = property on="Rev/Fwd" class="Clust (strict)"("Visible"=w338) -> ()  [unwired: 2 in, 2 out]
        n218 = property on="Test Ring" class="Ring (strict)"("Visible"=w338) -> ()  [unwired: 2 in, 2 out]
      }
      event "Listbox": Double Click {
        n219 = event-data() -> ("PlatMods.Shift"=w346:bool, "Row"=w348:i32)  [unwired: 1 in]
        n220 = case shown="True" w346 {
          tunnel: w348 -> [w352 _]
          tunnel: 1 -> [w351 _]
          frame False {
            n221 = property on="Listbox" class="LstBox (strict)"() -> ("Item Symbols"=w350:i32[])  [unwired: 2 in, 2 out]
            n222 = Replace Array Subset(array=w350, new element=w351, index=w352) -> (w349:i32[])
            n223 = property on="Listbox" class="LstBox (strict)"("Item Symbols"=w349) -> ()  [unwired: 2 in, 2 out]
          }
          frame True {
            w353 = 0 ("Top Row")
            n224 = property on="Listbox" class="LstBox (strict)"() -> ("Number of Rows"=w355:u32)  [unwired: 2 in, 2 out]
            n225 = Initialize Array(0, w355) -> (w354:i32[])
            n226 = property on="Listbox" class="LstBox (strict)"("Top Row"=w353, "Value"=w353, "Item Symbols"=w354) -> ()  [unwired: 2 in, 2 out]
          }
        }
      }
      event "Listbox": Key Down {
        n227 = event-data() -> ("VKey"=w359:T23)  [unwired: 1 in]
        n228 = case shown="\"Left\", \"Right\"" w359 {
          selector: w359 -> [w364 _]
          tunnel: eventvkey."Left" ("VKey") -> [w362 _]
          frame "Left", "Right" {
            n229 = Equal?(x=w362, y=w364) -> (x = y?=w363:bool)
            n230 = Select(t=0, s=w363, f=1) -> (s? t:f=w365:i32)
            n231 = property on="Listbox" class="LstBox (strict)"() -> ("Item Symbols"=w368:i32[])  [unwired: 2 in, 2 out]
            n232 = Replace Array Subset(array=w368, new element=w365, index="Listbox") -> (w367:i32[])
            n233 = property on="Listbox" class="LstBox (strict)"("Item Symbols"=w367) -> ()  [unwired: 2 in, 2 out]
          }
          frame Default {
          }
        }
      }
      event "DB Camera Config": Value Change {
        n234 = event-data() -> ("NewVal"=w372:bool)  [unwired: 1 in]
        n235 = case shown="False" w372 {
          tunnel: w371 -> [w381 _]
          tunnel: [w374 w392] -> w370
          tunnel: w369 -> [w373 w392]
          frame False {
            w388 = "Camera"
            w391 = FALSE ("Visible")
            n236 = local read "Camera Settings"() -> (w380:T1)
            n237 = Index Array(array=w381) -> (element=w384:cluster{string[]})  [unwired: 1 in]
            n238 = Unbundle(w380) -> ("Frame Rate"=w379:i32, "Compression"=w378:i32, "Size"=w382:u16)
            n239 = Unbundle(w384) -> (w383:string[])
            n240 = Index Array(array=w383, index=w382) -> (element=w377:string)
            n241 = call-poly <vilib>:"Write Key.vi"("section"=w388, "value"=w377, "key"="Size", "refnum"=w373) -> ("refnum out"=w390:T19)  [unwired: 2 in, 5 out]
            n242 = call-poly <vilib>:"Write Key.vi"("section"=w388, "value"=w379, "key"="FrameRate", "refnum"=w390) -> ("refnum out"=w389:T19)  [unwired: 1 in, 6 out]
            n243 = local write "DB Camera Config"(w391) -> ()
            n244 = property on="Camera Settings" class="Clust (strict)"("Visible"=w391) -> ()  [unwired: 2 in, 2 out]
            n245 = call-poly <vilib>:"Write Key.vi"("section"=w388, "value"=w378, "key"="Compression", "refnum"=w389) -> ("refnum out"=w375:T19)  [unwired: 1 in, 6 out]
            n246 = call <vilib>:"Close Config Data.vi"("refnum"=w375) -> ("file path"=w376:path)  [unwired: 2 in, 8 out]
            n247 = call <vilib>:"Open Config Data.vi"("configuration file path"=w376) -> ("refnum"=w374:T19)  [unwired: 8 in, 2 out]
          }
          frame True {
            n248 = property on="Camera Settings" class="Clust (strict)"("Visible"=TRUE) -> ()  [unwired: 2 in, 2 out]
          }
        }
      }
      event "Camera Settings": Value Change {
        n249 = event-data() -> ("NewVal"=w405:T1)  [unwired: 1 in]
        n250 = Index Array(array=w401) -> (element=w400:cluster{string[]})  [unwired: 1 in]
        n251 = Unbundle(w405) -> ("Frame Rate"=w396:i32, "Compression"=w395:i32, "Size"=w398:u16)
        n252 = Unbundle(w400) -> (w399:string[])
        n253 = Index Array(array=w399, index=w398) -> (element=w397:string)
        n254 = Format Into String(format string="%s   %dfps   %d%%", w397, w396, w395) -> (resulting string=w402:string)  [unwired: 2 in, 1 out]
        n255 = Build Array(w402) -> (w403:string[])
        n256 = property on="DB Camera Config" class="Bool (strict)"("Strings [4]"=w403) -> ()  [unwired: 2 in, 2 out]
      }
      event "Motor.Enable": Value Change {
        n257 = event-data() -> ("NewVal"=w411:bool)  [unwired: 1 in]
        n258 = Unbundle("Motor") -> ("Value"=w410:dbl)  [unwired: 1 out]
        n259 = Select(t=w410, s=w411, f=0.0) -> (s? t:f=w408:dbl)
        n260 = call <vilib>:"NT Write Number.vi"("Numeric"=w408, "Name"=w407) -> ()  [unwired: 9 in, 1 out]
      }
      event "Test Slider": Value Change {
        n261 = event-data() -> ("NewVal"=w414:dbl)  [unwired: 1 in]
        n262 = call <vilib>:"NT Write Number.vi"("Numeric"=w414, "Name"=w415) -> ()  [unwired: 9 in, 1 out]
      }
      event "On/Off": Value Change {
        n263 = event-data() -> ("NewVal"=w419:bool)  [unwired: 1 in]
        n264 = Boolean To (0,1)(Boolean=w419) -> (0, 1=w418:i16)
        n265 = call <vilib>:"NT Write Number.vi"("Numeric"=w418, "Name"=w417) -> ()  [unwired: 9 in, 1 out]
      }
      event "Rev/Fwd": Value Change {
        n266 = event-data() -> ("NewVal.Forward"=w427:bool, "NewVal.Reverse"=w426:bool)  [unwired: 1 in]
        n267 = Boolean To (0,1)(Boolean=w427) -> (0, 1=w423:i16)
        n268 = Boolean To (0,1)(Boolean=w426) -> (0, 1=w425:i16)
        n269 = Negate(x=w425) -> (-x=w424:i16)
        n270 = Add(x=w423, y=w424) -> (x+y=w422:i16)
        n271 = call <vilib>:"NT Write Number.vi"("Numeric"=w422, "Name"=w421) -> ()  [unwired: 9 in, 1 out]
      }
      event "Test Ring": Value Change {
        n272 = event-data() -> ("NewVal"=w431:u16)  [unwired: 1 in]
        n273 = property on="Test Ring" class="Ring (strict)"() -> ("Strings []"=w432:string[])  [unwired: 2 in, 2 out]
        n274 = Index Array(array=w432, index=w431) -> (element=w430:string)
        n275 = call <vilib>:"NT Write String.vi"("String"=w430, "Name"=w429) -> ()  [unwired: 9 in, 1 out]
      }
      event "Rec Mode": Value Change {
        # "Update globals for recording mode and path to read log from.\nClear when logging and let NetworkTables set path for vision to\nuse."
        n276 = event-data() -> ("NewVal"=w442:enum32{"Stop", "Record", "Playback"})  [unwired: 1 in]
        n277 = global write "WPI_DashboardLogging Global.vi" "Logging Filename"(path "") -> ()
        n278 = global write "WPI_DashboardLogging Global.vi" "Recording"(w442) -> ()
        n279 = case shown="\"Stop\", \"Record\"" w442 {
          tunnel: w441 -> [_ w444 w452]
          tunnel: [_ _ w451] -> w438
          tunnel: [_ _ w450] -> _
          tunnel: w436 -> [_ _ w448]
          tunnel: cluster{i32, i32} {-250, 170} -> [_ _ w447]
          tunnel: [_ _ T24 {"Image Size"=TRUE, "Image Type"=TRUE, "Pixel Value"=TRUE, "ROI Information"=TRUE, "Zoom Factor"=FALSE} ("Image Information Shown:All Elements")] -> w433
          tunnel: [_ _ TRUE ("Zoom Factor")] -> w434
          frame Default {
          }
          frame "Stop", "Record" {
            # "Place Window too"
            n280 = invoke class="VI" method="FP.Close"(reference=w444) -> (reference out=w443:refnum<vi>)  [unwired: 2 in, 2 out]
            n281 = invoke class="VI" method="Abort VI"(reference=w443) -> ()  [unwired: 2 in, 3 out]
          }
          frame "Playback" {
            n282 = call "Open Playback Panel.vi"("Offset"=w447, "DB VI Ref"=w448, "Playback in"=w452) -> ("Playback out"=w449:refnum<vi>)  [unwired: 8 in]
            n283 = register-events(w449) -> (reference out=w451:refnum<event-registration>, error out=w450:errorcluster)  [unwired: 2 in]
          }
        }
        n284 = property on="Image 2" class="ImageControl"("Image Information Shown"=w433, "Image Information Visible"=w434) -> ()  [unwired: 2 in, 2 out]
        n285 = call <vilib>:"WPI_DashboardNT Log FieldName Cache.vi"("Operation"=enum16{"Lookup/Add", "Index", "Clear"}."Clear") -> ()  [unwired: 8 in, 3 out]
      }
      event Panel Close {
        w453 = enum32{"Stop", "Record", "Playback"}."Stop" ("Rec Mode")
        n286 = event-data() -> ()  [unwired: 1 in, 4 out]
        n287 = local write "Rec Mode"(w453) -> ()
        n288 = global write "WPI_DashboardLogging Global.vi" "Recording"(w453) -> ()
      }
      event Panel Close {
        # "Abort playback window and ourself"
        n289 = event-data() -> ()  [unwired: 1 in, 4 out]
        n290 = invoke class="VI" method="FP.Close"(reference=w458) -> (reference out=w457:refnum<vi>)  [unwired: 2 in, 2 out]
        n291 = invoke class="VI" method="Abort VI"(reference=w457) -> (error out=w456:errorcluster)  [unwired: 2 in, 2 out]
        n292 = invoke class="VI" method="Abort VI"(error in=w456) -> ()  [unwired: 2 in, 3 out]
      }
    }
  }
  n293 = property on="On/Off" class="Bool (strict)"("Visible"=w25) -> ()  [unwired: 2 in, 2 out]
  n294 = property on="Motor" class="Clust (strict)"("Visible"=w25) -> ()  [unwired: 2 in, 2 out]
  n295 = property on="Progress" class="Clust (strict)"("Visible"=w25) -> ()  [unwired: 2 in, 2 out]
  n296 = property on="Test Ring" class="Ring (strict)"("Visible"=w25) -> ()  [unwired: 2 in, 2 out]
  n297 = property on="Rev/Fwd" class="Clust (strict)"("Visible"=w25) -> ()  [unwired: 2 in, 2 out]
  n298 = property on="Camera Settings" class="Clust (strict)"("Visible"=w25) -> ()  [unwired: 2 in, 2 out]
  n299 = local write "DB Camera Config"(w25) -> ()
  n300 = global write "WPI_DashboardLogging Global.vi" "Recording"(w10) -> ()
  n301 = local write "Rec Mode"(w10) -> ()
  n302 = while {
    stop <- FALSE stop-if-true
    n303 = Wait Until Next ms Multiple(millisecond multiple=u32 100) -> ()  [unwired: 1 out]
    n304 = call <vilib>:"SD Write Number.vi"("Numeric"="Routine selected", "Name"="Routine selected") -> ()  [unwired: 8 in, 2 out]
    n305 = property on="Routine selected" class="Ring (strict)"("Strings []"="Auton Routine Names") -> ()  [unwired: 2 in, 2 out]
  }
